vi "Init.vi"(8 "error in":errorcluster, 10 "Type":variant, 11 "Combo Box in":refnum<class "Combo Box.lvclass">) -> (0 "error out":errorcluster, 3 "Combo Box out":refnum<class "Combo Box.lvclass">)   [LabVIEW 2024, in "SourceGrid.lvlib" / "Combo Box.lvclass"]
uses:
  Combo Box.lvclass
  Combo Box.lvclass/Combo Box.ctl
  D:/git/Sourcegrid-LabVIEW/dll/SourceGrid.dll
  dll/SourceGrid.dll
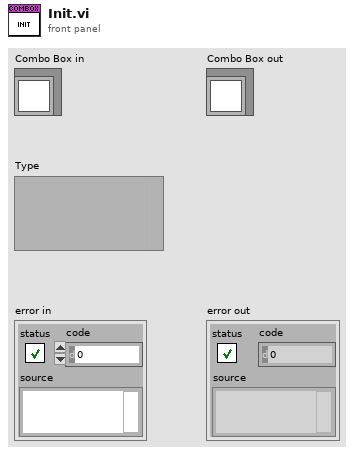
[diagram p1: front panel]
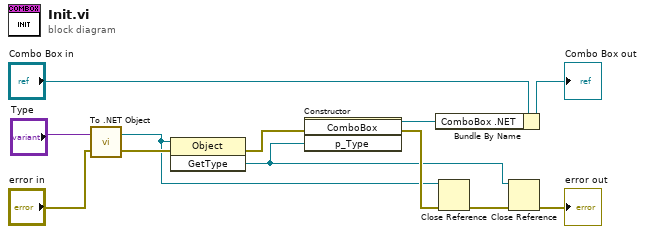
[diagram p0: block diagram]
diagram:
  n1 = call <vilib>:"To .NET Object.vi"("error in (no error)"="error in", "anything"="Type") -> ("error out"=w6:errorcluster, ".NET object"=w3:refnum<k24>)
  n2 = invoke class="Object" method="GetType"(reference=w3, error in=w6) -> (error out=w5:errorcluster, "GetType"=w1:refnum<k24>)  [unwired: 1 in, 1 out]
  n3 = constructor class="ComboBox"(error in=w5, "p_Type"=w1) -> (reference out=w7:refnum<k24>, error out=w9:errorcluster)  [unwired: 2 in, 2 out]
  n4 = Bundle By Name(cluster="Combo Box in", "ComboBox .NET"=w7) -> (→"Combo Box out":refnum<class "Combo Box.lvclass">)
  n5 = Close Reference(reference=w3, error in (no error)=w9) -> (error out=w4:errorcluster)
  n6 = Close Reference(reference=w1, error in (no error)=w4) -> (error out=→"error out":errorcluster)
